vi "_Parse IEM List I32 Result.vi"(8 "error in (no error)":errorcluster, 10 "Input String":string, 11 "VISA resource name":refnum<visa-resource-name>) -> (0 "error out":errorcluster, 1 "Results":T1(array[cluster]), 2 "Reliability":i32, 3 "VISA resource name out":refnum<visa-resource-name>)   [LabVIEW 2020, in "Rohde&Schwarz CMXP NR FR2 Measurement.lvlib"]
uses:
  <instrlib>/Rohde&Schwarz CMXP NR FR2 Measurement/Rohde&Schwarz CMXP NR FR2 Measurement.lvlib
  <instrlib>/Rohde&Schwarz CMXP NR FR2 Measurement/Private/rsidr_core.llb/rsidr_core.lvlib
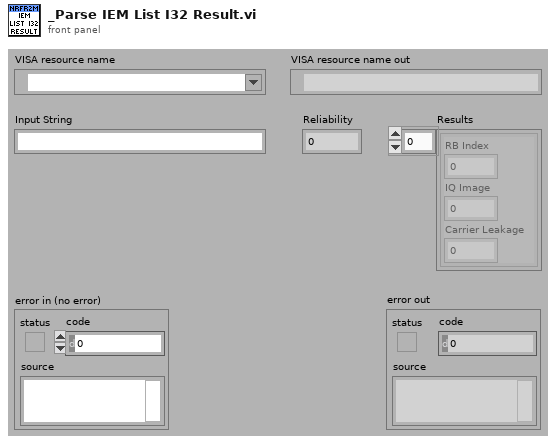
[diagram p1: front panel]
types:
  T1 = cluster{"RB Index":i32, "IQ Image":i32, "Carrier Leakage":i32}[]
  T2 = cluster{"RB Index":i32, "IQ Image":i32, "Carrier Leakage":i32}
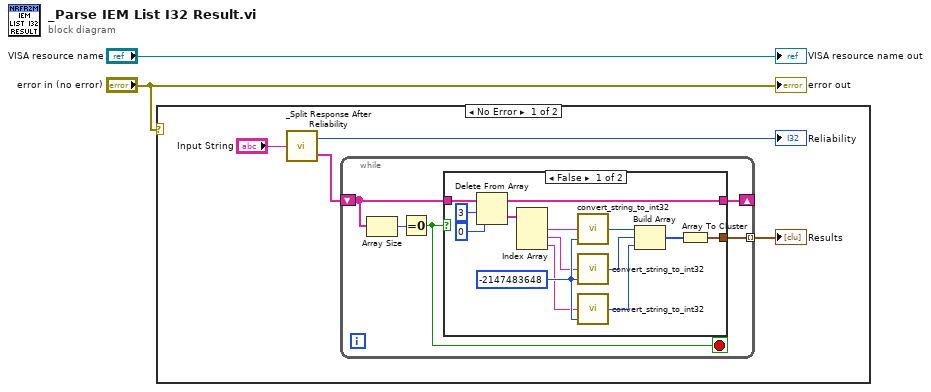
[diagram p0: block diagram]
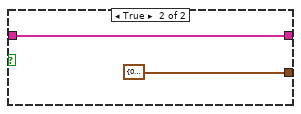
[diagram p2: hidden frame]
diagram:
  n1 = case shown="No Error" "error in (no error)" {
    frame No Error {
      n2 = call <instrlib>:"_Split Response After Reliability.vi"("Input String"="Input String") -> ("Response out"=w3:string[], "Reliability out"=→"Reliability":i32)
      n3 = while {
        shift-right: [w8] -> _
        shift-left: w3 -> [w9]
        tunnel: [w7] -> w4 mode=indexing
        stop <- w10 stop-if-true
        n4 = Array Size(array=w9) -> (size(s)=w11:i32)
        n5 = Equal To 0?(x=w11) -> (x = 0?=w10:bool)
        n6 = case shown="False" w10 {
          tunnel: w9 -> [w25 w27]
          tunnel: [w22 w27] -> w8
          tunnel: [w12 T2 {"RB Index"=0, "IQ Image"=0, "Carrier Leakage"=0} ("RB Index Result")] -> w7
          frame False {
            w20 = -2147483648
            n7 = Delete From Array(array=w25, length=3, index=0) -> (deleted portion=w21:string[], array with subset deleted=w22:string[])
            n8 = Index Array(array=w21) -> (element #1=w19:string, element #2=w17:string, element #3=w18:string)  [unwired: 3 in]
            n9 = call <instrlib>:"convert_string_to_int32.vi"("default (0)"=w20, "String in"=w19) -> ("int32 value out"=w16:i32)  [unwired: 3 in]
            n10 = call <instrlib>:"convert_string_to_int32.vi"("default (0)"=w20, "String in"=w17) -> ("int32 value out"=w14:i32)  [unwired: 3 in]
            n11 = call <instrlib>:"convert_string_to_int32.vi"("default (0)"=w20, "String in"=w18) -> ("int32 value out"=w15:i32)  [unwired: 3 in]
            n12 = Build Array(w16, w14, w15) -> (w13:i32[])
            n13 = Array To Cluster(array=w13) -> (cluster=w12:cluster{"[0]":i32, "[1]":i32, "[2]":i32})
          }
          frame True {
          }
        }
      }
      "Results" <- w4
    }
    frame Error {
    }
  }
  "VISA resource name out" <- "VISA resource name"
  "error out" <- "error in (no error)"
